vi "VI Server_TREE_Symbols_Colors_CLEAR.vi"(7 "Label":string, 8 "error in":errorcluster, 9 "Tree.Ref":refnum<vi>, 11 "VI Server.RefsCluster":T1) -> (0 "error out":errorcluster, 1 "Tree.Ref.DUP":refnum<vi>, 3 "VI Server.RefsCluster.DUP":T1)   [LabVIEW 2020]
uses:
  VI Server_TypeDefs/VI Server_RefsCluster.ctl
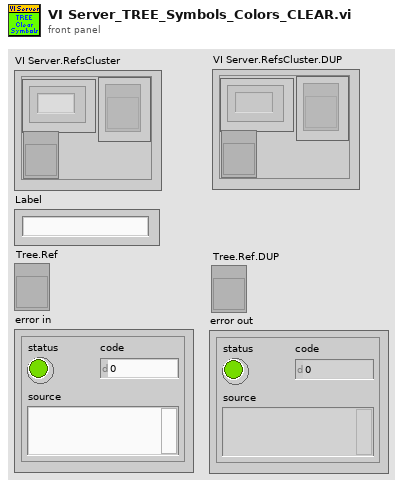
[diagram p1: front panel]
types:
  T1 = typedef "VI Server_RefsCluster.ctl" = cluster{"Labels":string[], "Refs":refnum<vi>[], "VI Ref":refnum<vi>}
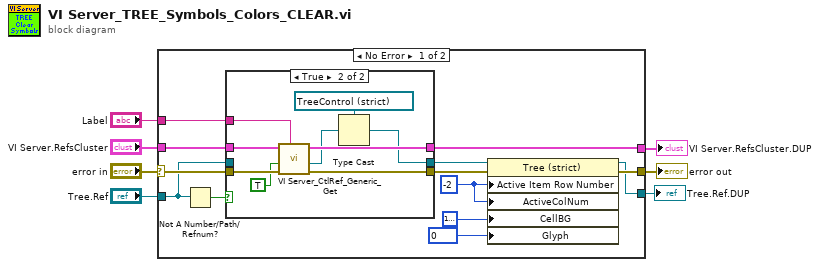
[diagram p0: block diagram]
diagram:
  n1 = case shown="No Error" "error in" {
    selector: "error in" -> [w20 w34]
    tunnel: [w13 w34] -> w6
    tunnel: "VI Server.RefsCluster" -> [w19 w33]
    tunnel: [w18 w33] -> w4
    tunnel: "Label" -> [w17 _]
    tunnel: [w9 _] -> w1
    tunnel: "Tree.Ref" -> [w15 _]
    frame No Error {
      w12 = -2 ("Active Item:Row Number")
      n2 = Not A Number/Path/Refnum?(number/path/refnum=w15) -> (NaN/Path/Refnum?=w16:bool)
      n3 = case shown="True" w16 {
        tunnel: w20 -> [w23 w32]
        tunnel: w19 -> [w21 w31]
        tunnel: [w21 w30] -> w18
        tunnel: w17 -> [_ w29]
        tunnel: [w22 w27] -> w10
        tunnel: [w23 w26] -> w14
        tunnel: w15 -> [w22 _]
        frame False {
        }
        frame True {
          n4 = call "VI Server_CtlRef_Generic_Get.vi"("Control.Label"=w29, "error in"=w32, "SingleInstance"=TRUE, "VI Server.RefsCluster"=w31) -> ("error out"=w26:errorcluster, "Control.Ref.Generic"=w28:refnum<vi>, "VI Server.RefsCluster.DUP"=w30:T1)  [unwired: 5 in]
          n5 = Type Cast(type=refnum<vi> refnum ("Test.Tree"), x=w28) -> (*(type *) &x=w27:refnum<vi>)
        }
      }
      n6 = property on="Property Node" class="Tree (strict)"(reference=w10, error in=w14, "Active Item Row Number"=w12, "ActiveColNum"=w12, "CellBG"=u32 16777226, "Glyph"=0) -> (reference out=w9:refnum<vi>, error out=w13:errorcluster)
    }
    frame Error {
    }
  }
  "VI Server.RefsCluster.DUP" <- w4
  "error out" <- w6
  "Tree.Ref.DUP" <- w1
